vi "Create User Event - Stop.vi"(8 "에러 입력(에러 없음)":errorcluster) -> (0 "에러 출력":errorcluster, 2 "사용자 이벤트 - 정지":refnum<user-event>, 3 "이벤트 등록 참조 번호 출력":refnum<event-registration>)   [LabVIEW 2020]
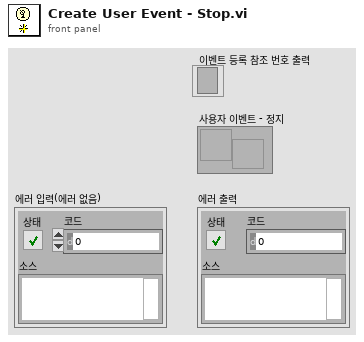
[diagram p1: front panel]
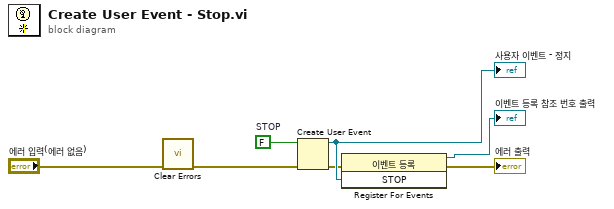
[diagram p0: block diagram]
diagram:
  w2 = FALSE  # STOP
  n1 = call <vilib>:"Clear Errors.vi"("error in (no error)"="에러 입력(에러 없음)") -> ("error out"=w1:errorcluster)  [unwired: 5 in, 1 out]
  n2 = Create User Event(user event datatype=w2, error in=w1) -> (user event=w7:refnum<user-event>, error out=w3:errorcluster)
  "사용자 이벤트 - 정지" <- w7
  n3 = register-events(error in=w3, w7) -> (reference out=→"이벤트 등록 참조 번호 출력":refnum<event-registration>, error out=→"에러 출력":errorcluster)  [unwired: 1 in]
